vi "AKD Operational Mode.vi"(0 "connection ID":refnum<k5>, 7 "Operational Mode":u16(ring) items=["Current (torque) Operation Mode", "Velocity Operation Mode", "Position Operation Mode"], 11 "error in":errorcluster) -> (4 "TCP Refnum":refnum<k5>, 15 "error out":errorcluster)   [LabVIEW 2019]
uses:
  MODBUS/NI Modbus.llb/MB Ethernet Master Query Write Multiple Registers (poly).vi
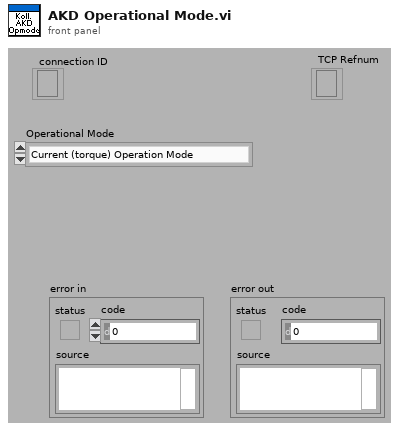
[diagram p1: front panel]
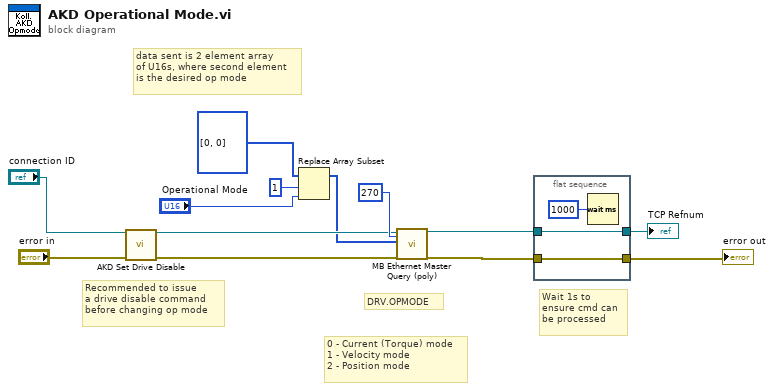
[diagram p0: block diagram]
diagram:
  # "Wait 1s to \nensure cmd can\nbe processed"
  # "0 - Current (Torque) mode\n1 - Velocity mode\n2 - Position mode"
  # "data sent is 2 element array\nof U16s, where second element\nis the desired op mode"
  # "Recommended to issue\na drive disable command\nbefore changing op mode"
  # "DRV.OPMODE"
  n1 = call "AKD Set Drive Disable.vi"("connection ID"="connection ID", "error in"="error in") -> ("TCP Refnum"=w9:refnum<k5>, "error out"=w11:errorcluster)  [unwired: 12 in]
  n2 = Replace Array Subset(array=u16[] [0, 0], new element="Operational Mode", index=1) -> (w8:u16[])
  n3 = call-poly "MB Ethernet Master Query (poly).vi"("TCP Connection Refnum in"=w9, "Starting Address"=u16 270, "Registers"=w8, "error in"=w11) -> ("TCP Connection Refnum (dup)"=w3:refnum<k5>, "error out"=w4:errorcluster)  [unwired: 13 in, 1 out]
  n4 = flat-sequence {
    tunnel: [w15] -> w2
    tunnel: w3 -> [w15]
    tunnel: w4 -> [w14]
    tunnel: [w14] -> w1
    frame #0 {
      n5 = Wait (ms)(milliseconds to wait=u32 1000) -> ()  [unwired: 1 out]
    }
  }
  "error out" <- w1
  "TCP Refnum" <- w2
